vi "niScope Close.vi"(0 "instrument handle":refnum<k15>, 11 "error in":errorcluster) -> (15 "error out":errorcluster)   [LabVIEW 2020]
doc: "Performs the following actions:\n\n-Closes the instrument I/O session.\n\n-Destroys the IVI session and all of its properties.\n\n-Deallocates any memory resources used by the IVI session.\n\nCall this VI when you are finished using an instrument driver session."
uses:
  niScope_32.dll
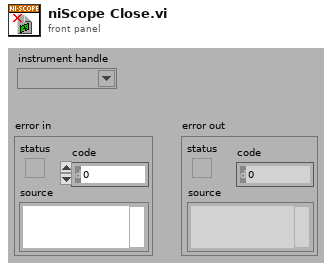
[diagram p1: front panel]
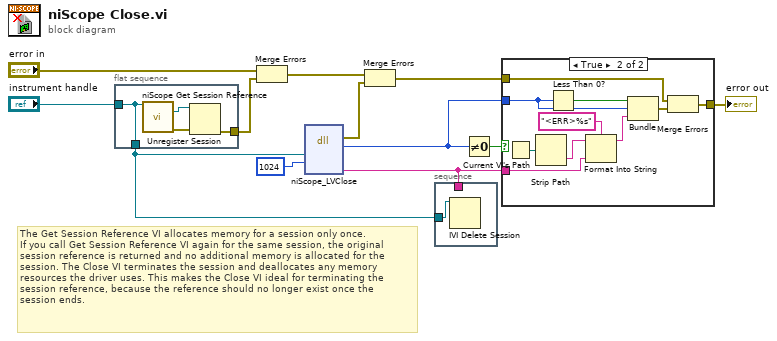
[diagram p0: block diagram]
diagram:
  # "The Get Session Reference VI allocates memory for a session only once.  \nIf you call Get Session Reference VI again for the same session, the original \nsession reference is returned and no additional memory is allocated for the \nsession. The Close VI terminates the session and deallocates any memory \nresources the driver uses. This makes the Close VI ideal for terminating the \nsession reference, because the reference should no longer exist once the \nsession ends."
  n1 = flat-sequence {
    tunnel: "instrument handle" -> [w13]
    tunnel: [w16] -> w10
    tunnel: [w13] -> w4
    frame #0 {
      n2 = call "niScope Get Session Reference.vi"("instrument handle"=w13) -> ("session reference"=w14:refnum<k20>, "error out"=w15:errorcluster)  [unwired: 12 in, 1 out]
      n3 = Unregister Session(8:w15, 11:w14) -> (0:w16:errorcluster)
    }
  }
  n4 = Merge Errors("error in", w10) -> (w3:errorcluster)
  n5 = dll-call lib="niScope_*.*" fn="niScope_LVClose"("instrument handle"=w4, "buffer size"=1024) -> (error out=w2:errorcluster, "status"=w5:i32, "error buffer"=w7:string)  [unwired: 6 in, 1 out]
  n6 = Merge Errors(w3, w2) -> (w1:errorcluster)
  n7 = stacked-sequence {
    tunnel: w4 -> [w17]
    tunnel: w7 -> [_]
    frame #0 {
      n8 = IVI Delete Session(11:w17) -> ()
    }
  }
  n9 = Not Equal To 0?(x=w5) -> (x != 0?=w6:bool)
  n10 = case shown="True" w6 {
    tunnel: w5 -> [_ w23]
    tunnel: w7 -> [_ w26]
    tunnel: [w18 w19] -> w12
    tunnel: w1 -> [w18 w21]
    frame False {
    }
    frame True {
      n11 = Current VI's Path() -> (path=w28:path)
      n12 = Strip Path(path=w28) -> (name=w27:string)  [unwired: 1 out]
      n13 = Less Than 0?(x=w23) -> (x < 0?=w22:bool)
      n14 = Format Into String(format string="<ERR>%s" ("Format String"), initial string=w27, w26) -> (resulting string=w24:string)  [unwired: 1 in, 1 out]
      n15 = Bundle(w22, "status"=w23, w24) -> (w20:cluster{bool, "status":i32, string})  [unwired: 1 in]
      n16 = Merge Errors(w21, w20) -> (w19:errorcluster)
    }
  }
  "error out" <- w12
